vi "CurrentOutput_flt.vi"(7 "y scaled":dbl, 9 "array":dbl[][](array[numeric]), 10 "Z Input":dbl, 11 "X Input":dbl) -> (0 "Origin":dbl, 1 "FW":dbl, 2 "FH":dbl, 3 "Current Out (pA)":dbl, 4 "Zread":dbl)   [LabVIEW 2019]
uses:
  <vilib>/ptbypt/NI_PtbyPt.lvlib
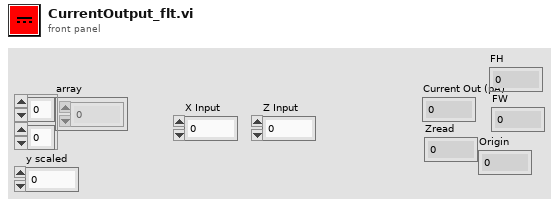
[diagram p1: front panel]
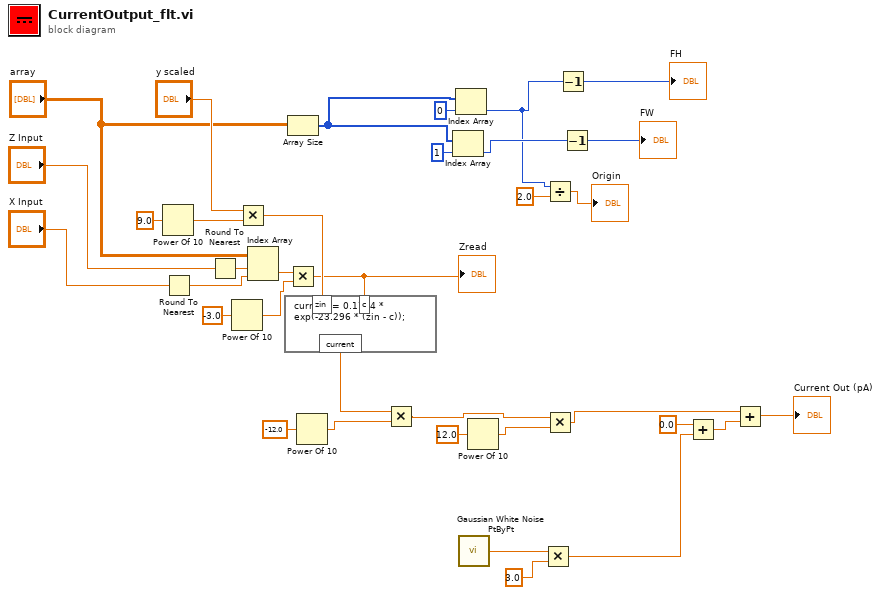
[diagram p0: block diagram]
diagram:
  n1 = Power Of 10(x=9.0) -> (10^x=w31:dbl)
  n2 = Round To Nearest(number="X Input") -> (nearest integer value=w25:dbl)
  n3 = Round To Nearest(number="Z Input") -> (nearest integer value=w33:dbl)
  n4 = Power Of 10(x=-3.0) -> (10^x=w27:dbl)
  n5 = Multiply(x="y scaled", y=w31) -> (x*y=w29:dbl)
  n6 = Index Array(array="array", index (row)=w33, index (col)=w25) -> (element=w22:dbl)
  n7 = Array Size(array="array") -> (size(s)=w17:i32[])
  n8 = Multiply(x=w22, y=w27) -> (x*y=w26:dbl)
  "Zread" <- w26
  n9 = formula code="current = 0.1714 * exp(-23.296 * (zin - c));"("zin"=w29, "c"=w26) -> ("current"=w32:dbl)
  n10 = Power Of 10(x=-12.0) -> (10^x=w35:dbl)
  n11 = Multiply(x=w32, y=w35) -> (x*y=w3:dbl)
  n12 = Index Array(array=w17, index=1) -> (element=w16:i32)
  n13 = Index Array(array=w17, index=0) -> (element=w14:i32)
  n14 = call <vilib>:"Gaussian White Noise PtByPt.vi"() -> ("Gaussian white noise"=w7:dbl)  [unwired: 3 in]
  n15 = Power Of 10(x=12.0) -> (10^x=w10:dbl)
  n16 = Multiply(x=w7, y=3.0) -> (x*y=w4:dbl)
  n17 = Divide(x=w14, y=2.0) -> (x/y=→"Origin":dbl)
  n18 = Multiply(x=w3, y=w10) -> (x*y=w8:dbl)
  n19 = Decrement(x=w14) -> (x-1=→"FH":i32)
  n20 = Decrement(x=w16) -> (x-1=→"FW":i32)
  n21 = Add(x=0.0, y=w4) -> (x+y=w5:dbl)
  n22 = Add(x=w8, y=w5) -> (x+y=→"Current Out (pA)":dbl)
